vi "CRC16.vi"(11 "Data in":string) -> (3 "CRC-16":u16 format="%04x")   [LabVIEW 2021, in "Config.lvlib"]
doc: "Calculates the 16-bit CRC using the CRC-16/BUYPASS algorithm."
uses:
  Config.lvlib
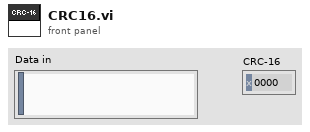
[diagram p1: front panel]
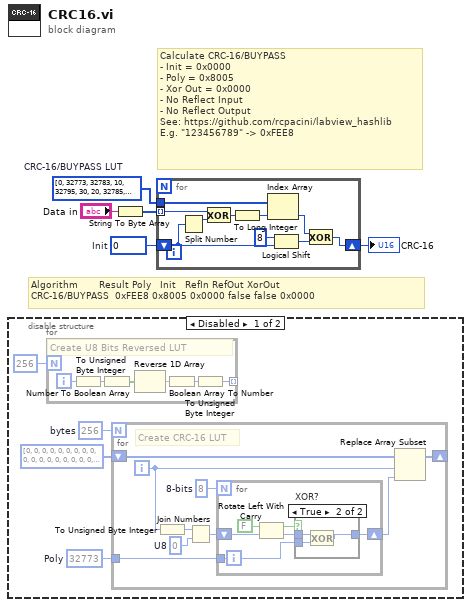
[diagram p0: block diagram]
diagram:
  w1 = u16[] [0, 32773, 32783, 10, 32795, 30, 20, 32785, 32819, 54, 60, 32825, 40, 32813, 32807, 34, 32867, 102, 108, 32873, 120, 32893, 32887, 114, 80, 32853, 32863, 90, 32843, 78, 68, 32833, 32963, 198, 204, 32969, 216, 32989, 32983, 210, 240, 33013, 33023, 250, 33003, 238, 228, 32993, 160, 32933, 32943, 170, 32955, 190, 180, 32945, 32915, 150, 156, 32921, 136, 32909, 32903, 130, 33155, 390, 396, 33161, 408, 33181, 33175, 402, 432, 33205, 33215, 442, 33195, 430, 420, 33185, 480, 33253, 33263, 490, 33275, 510, 500, 33265, 33235, 470, 476, 33241, 456, 33229, 33223, 450, 320, 33093, 33103, 330, 33115, 350, 340, 33105, 33139, 374, 380, 33145, 360, 33133, 33127, 354, 33059, 294, 300, 33065, 312, 33085, 33079, 306, 272, 33045, 33055, 282, 33035, 270, 260, 33025, 33539, 774, 780, 33545, 792, 33565, 33559, 786, 816, 33589, 33599, 826, 33579, 814, 804, 33569, 864, 33637, 33647, 874, 33659, 894, 884, 33649, 33619, 854, 860, 33625, 840, 33613, 33607, 834, 960, 33733, 33743, 970, 33755, 990, 980, 33745, 33779, 1014, 1020, 33785, 1000, 33773, 33767, 994, 33699, 934, 940, 33705, 952, 33725, 33719, 946, 912, 33685, 33695, 922, 33675, 910, 900, 33665, 640, 33413, 33423, 650, 33435, 670, 660, 33425, 33459, 694, 700, 33465, 680, 33453, 33447, 674, 33507, 742, 748, 33513, 760, 33533, 33527, 754, 720, 33493, 33503, 730, 33483, 718, 708, 33473, 33347, 582, 588, 33353, 600, 33373, 33367, 594, 624, 33397, 33407, 634, 33387, 622, 612, 33377, 544, 33317, 33327, 554, 33339, 574, 564, 33329, 33299, 534, 540, 33305, 520, 33293, 33287, 514]  # CRC-16/BUYPASS LUT
  w5 = u16 0  # Init
  # "Calculate CRC-16/BUYPASS\n- Init = 0x0000\n- Poly = 0x8005\n- Xor Out = 0x0000\n- No Reflect Input\n- No Reflect Output\nSee: https://github.com/rcpacini/labview_hashlib\nE.g. \"123456789\" -> 0xFEE8"
  # "Algorithm       Result Poly   Init   RefIn RefOut XorOut\nCRC-16/BUYPASS  0xFEE8 0x8005 0x0000 false false 0x0000"
  n1 = disable-structure shown="Disabled" {
    frame Disabled {
      w7 = u16 32773  # Poly
      w8 = 256  # bytes
      n2 = for {
        N: 256 -> [_]
        tunnel: [w29] -> _ mode=indexing
        i -> [w34]
        # "Create U8 Bits Reversed LUT"
        n3 = To Unsigned Byte Integer(number=w34) -> (unsigned 8bit integer=w33:u8)
        n4 = Number To Boolean Array(number=w33) -> (Boolean array=w32:bool[])
        n5 = Reverse 1D Array(array=w32) -> (reversed array=w31:bool[])
        n6 = Boolean Array To Number(Boolean array=w31) -> (number=w30:u32)
        n7 = To Unsigned Byte Integer(number=w30) -> (unsigned 8bit integer=w29:u8)
      }
      n8 = for {
        N: w8 -> [_]
        tunnel: w7 -> [w15]
        shift-right: [w11] -> _
        shift-left: u16[] [0, 0, 0, 0, 0, 0, 0, 0, 0, 0, 0, 0, 0, 0, 0, 0, 0, 0, 0, 0, 0, 0, 0, 0, 0, 0, 0, 0, 0, 0, 0, 0, 0, 0, 0, 0, 0, 0, 0, 0, 0, 0, 0, 0, 0, 0, 0, 0, 0, 0, 0, 0, 0, 0, 0, 0, 0, 0, 0, 0, 0, 0, 0, 0, 0, 0, 0, 0, 0, 0, 0, 0, 0, 0, 0, 0, 0, 0, 0, 0, 0, 0, 0, 0, 0, 0, 0, 0, 0, 0, 0, 0, 0, 0, 0, 0, 0, 0, 0, 0, 0, 0, 0, 0, 0, 0, 0, 0, 0, 0, 0, 0, 0, 0, 0, 0, 0, 0, 0, 0, 0, 0, 0, 0, 0, 0, 0, 0, 0, 0, 0, 0, 0, 0, 0, 0, 0, 0, 0, 0, 0, 0, 0, 0, 0, 0, 0, 0, 0, 0, 0, 0, 0, 0, 0, 0, 0, 0, 0, 0, 0, 0, 0, 0, 0, 0, 0, 0, 0, 0, 0, 0, 0, 0, 0, 0, 0, 0, 0, 0, 0, 0, 0, 0, 0, 0, 0, 0, 0, 0, 0, 0, 0, 0, 0, 0, 0, 0, 0, 0, 0, 0, 0, 0, 0, 0, 0, 0, 0, 0, 0, 0, 0, 0, 0, 0, 0, 0, 0, 0, 0, 0, 0, 0, 0, 0, 0, 0, 0, 0, 0, 0, 0, 0, 0, 0, 0, 0, 0, 0, 0, 0, 0, 0, 0, 0, 0, 0, 0, 0, 0, 0, 0, 0, 0, 0] -> [w14]
        i -> [w13]
        w17 = 8  # 8-bits
        w18 = u8 0  # U8
        # "Create CRC-16 LUT"
        n9 = To Unsigned Byte Integer(number=w13) -> (unsigned 8bit integer=w10:u8)
        n10 = Join Numbers(hi=w10, lo=w18) -> ((hi.lo)=w16:u16)
        n11 = for {
          N: w17 -> [_]
          shift-right: [w20] -> w12
          shift-left: w16 -> [w24]
          tunnel: w15 -> [w21]
          n12 = Rotate Left With Carry(2:w24, 3:FALSE ("carry")) -> (0:w22:u16, 1:w19:bool)
          n13 = case "XOR?" shown="True" w19 {
            tunnel: w22 -> [w25 w28]
            tunnel: w21 -> [_ w27]
            tunnel: [w25 w26] -> w20
            frame False {
            }
            frame True {
              n14 = Exclusive Or(1:w27, 2:w28) -> (0:w26:u16)
            }
          }
        }
        n15 = Replace Array Subset(array=w14, new element=w12, index=w13) -> (w11:u16[])
      }
    }
    frame Enabled {
    }
  }
  n16 = String To Byte Array(string="Data in") -> (unsigned byte array=w3:u8[])
  n17 = for {
    shift-right: [w36] -> w2
    shift-left: w5 -> [w40]
    tunnel: w3 -> [w35] mode=indexing
    tunnel: w1 -> [w41]
    n18 = Split Number(x=w40) -> (hi(x)=w44:u8)  [unwired: 1 out]
    n19 = Exclusive Or(1:w44, 2:w35) -> (0:w43:u8)
    n20 = To Long Integer(number=w43) -> (32bit integer=w42:i32)
    n21 = Index Array(array=w41, index=w42) -> (element=w37:u16)
    n22 = Logical Shift(y=i16 8, x=w40) -> (x << y=w38:u16)
    n23 = Exclusive Or(1:w38, 2:w37) -> (0:w36:u16)
  }
  "CRC-16" <- w2
